vi "Read Scalar U8.vi"(8 "error in (no error)":errorcluster, 11 "pointer in":u64) -> (0 "error out":errorcluster, 2 "value":u8, 3 "pointer out":u64)   [LabVIEW 2013, in "Linux RT IPC.Shared Memory.lvlib"]
uses:
  Linux RT IPC.Shared Memory.lvlib
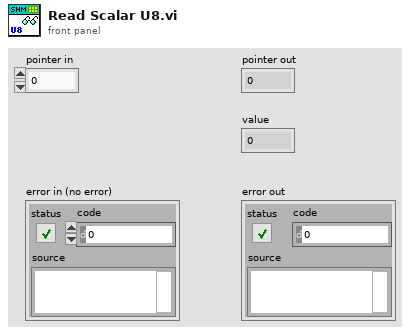
[diagram p1: front panel]
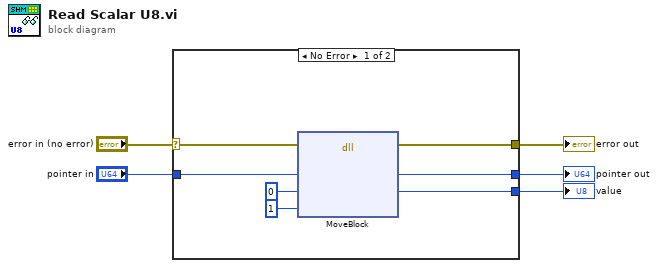
[diagram p0: block diagram]
diagram:
  n1 = case shown="No Error" "error in (no error)" {
    selector: "error in (no error)" -> [w10 w14]
    tunnel: [w9 w14] -> w5
    tunnel: "pointer in" -> [w7 w13]
    tunnel: [w8 w13] -> w2
    tunnel: [w6 _] -> w1
    frame No Error {
      n2 = dll-call lib="LabVIEW" fn="MoveBlock"(error in=w10, "pointer"=w7, "data"=u8 0, "size"=u64 1) -> (error out=w9:errorcluster, "pointer"=w8:u64, "data"=w6:u8)  [unwired: 4 in, 1 out]
    }
    frame Error {
    }
  }
  "error out" <- w5
  "pointer out" <- w2
  "value" <- w1
